vi "z_opti_rnd.vi"(0 "IP address":string="172.24.192.135", 1 "range[nm]":dbl, 3 "n":i32, 5 "Axis":string(combo), 7 "rand[t] seq [f]":bool, 9 "data":refnum<queue>, 11 "cam":refnum<queue>, 12 "error in (no error)":errorcluster) -> (4 "X":dbl[](array[numeric]), 6 "Y":dbl[](array[numeric]), 10 "Best Gaussian Fit":dbl[](array[numeric]), 14 "error out":errorcluster, 15 "center":dbl)   [LabVIEW 2017]
uses:
  <vilib>/gmath/NumericalOptimization/Nonlinear Curve Fit LM.vi
  <vilib>/gmath/NI_Gmath.lvlib
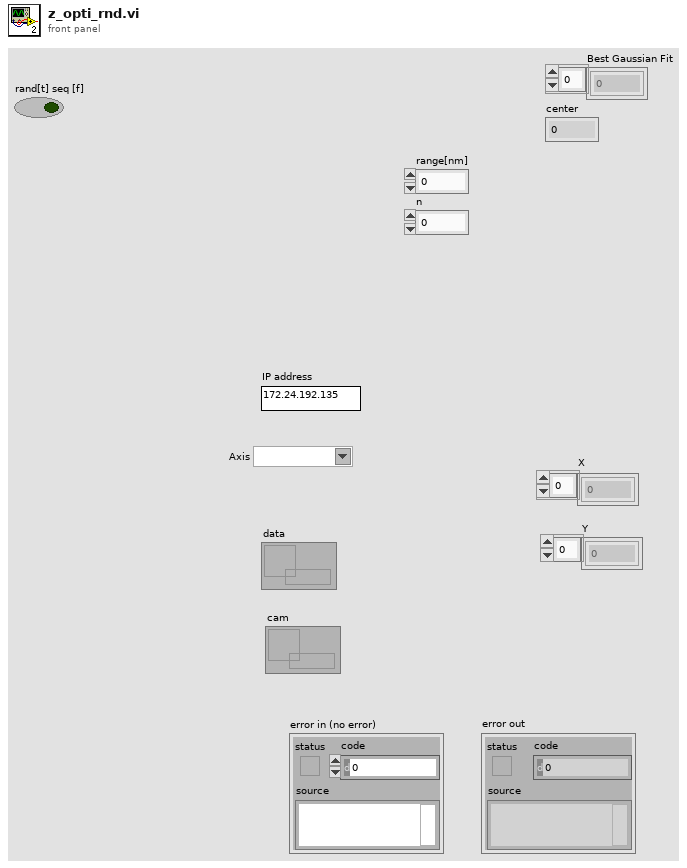
[diagram p1: front panel]
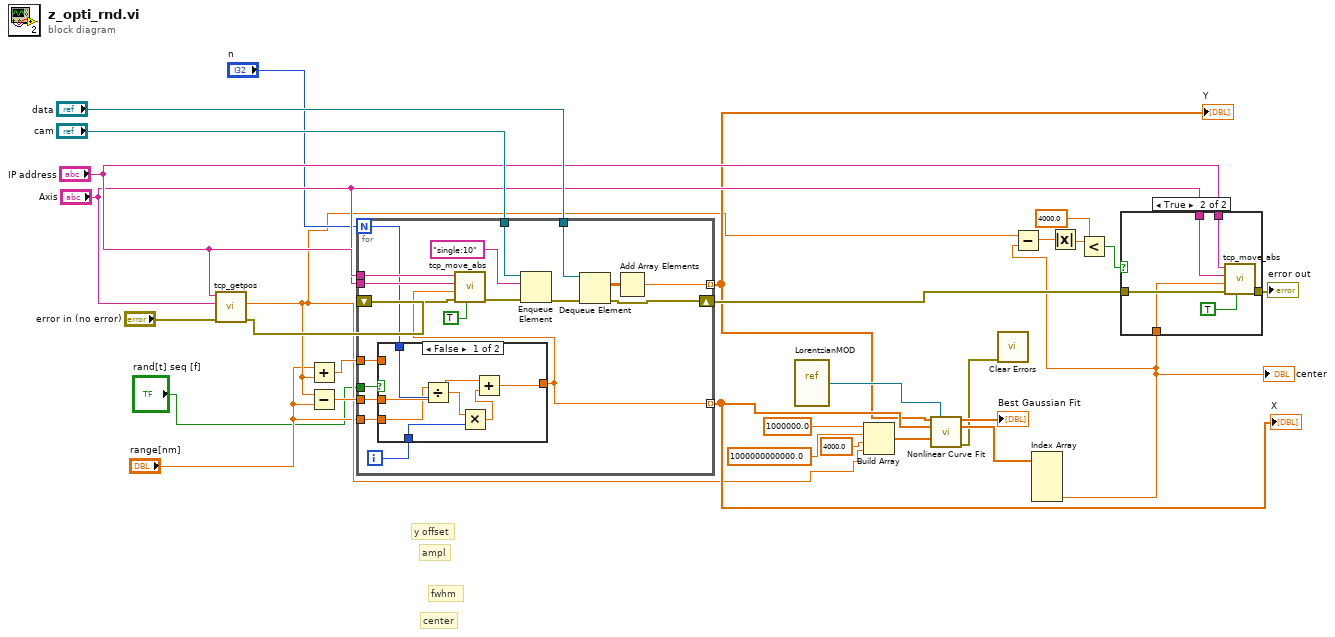
[diagram p0: block diagram]
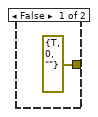
[diagram p2: hidden frame]
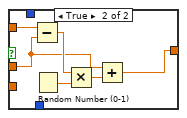
[diagram p3: hidden frame]
diagram:
  # "fwhm"
  # "ampl"
  # "center"
  # "y offset"
  n1 = call "tcp_getpos.vi"("error in (no error)"="error in (no error)", "Axis"="Axis", "IP address"="IP address") -> ("error out"=w24:errorcluster, "position"=w7:dbl)  [unwired: 6 in, 1 out]
  n2 = Add(x="range[nm]", y=w7) -> (x+y=w21:dbl)
  n3 = Subtract(x=w7, y="range[nm]") -> (x-y=w20:dbl)
  n4 = for {
    N: "n" -> [w32]
    tunnel: "Axis" -> [w48]
    tunnel: "IP address" -> [w47]
    tunnel: "cam" -> [w43]
    tunnel: "data" -> [w44]
    tunnel: [w39] -> w12 mode=indexing
    shift-right: [w37] -> w23
    shift-left: w24 -> [w38]
    tunnel: w21 -> [w36]
    tunnel: w20 -> [w35]
    tunnel: [w34] -> w17 mode=indexing
    tunnel: "range[nm]" -> [w31]
    tunnel: "rand[t] seq [f]" -> [w30]
    i -> [w33]
    n5 = case shown="False" w30 {
      tunnel: w36 -> [_ w58]
      tunnel: w35 -> [w55 w57]
      tunnel: [w54 w56] -> w34
      tunnel: w33 -> [w51 _]
      tunnel: w32 -> [w53 _]
      tunnel: w31 -> [w49 _]
      frame False {
        n6 = Divide(x=w49, y=w53) -> (x/y=w52:dbl)
        n7 = Multiply(x=w52, y=w51) -> (x*y=w50:dbl)
        n8 = Add(x=w55, y=w50) -> (x+y=w54:dbl)
      }
      frame True {
        n9 = Subtract(x=w58, y=w57) -> (x-y=w61:dbl)
        n10 = Random Number (0-1)() -> (number: 0 to 1=w60:dbl)
        n11 = Multiply(x=w61, y=w60) -> (x*y=w59:dbl)
        n12 = Add(x=w57, y=w59) -> (x+y=w56:dbl)
      }
    }
    n13 = call "tcp_move_abs.vi"("wait4motiondone"=TRUE, "error in (no error)"=w38, "destination nm/u°"=w34, "Axis"=w48, "IP address"=w47) -> ("error out"=w46:errorcluster)  [unwired: 4 in, 2 out]
    n14 = Enqueue Element(queue=w43, element="single:10", error in (no error)=w46) -> (error out=w45:errorcluster)  [unwired: 1 in, 2 out]
    n15 = Dequeue Element(queue=w44, error in (no error)=w45) -> (element=w40:dbl[][], error out=w37:errorcluster)  [unwired: 1 in, 2 out]
    n16 = Add Array Elements(numeric array=w40) -> (sum=w39:dbl)
  }
  "Y" <- w12
  "X" <- w17
  n17 = vi-ref "LorentzianMOD.vi"() -> (w18:refnum<vi>)
  n18 = Build Array(1000000.0 ("element"), 1000000000000.0 ("element"), 4000.0 ("element"), w7) -> (w14:dbl[])
  n19 = call-poly <vilib>:"Nonlinear Curve Fit.vi"("Y"=w12, "f(x,a)"=w18, "X"=w17, "initial parameters"=w14) -> ("best nonlinear fit"=→"Best Gaussian Fit":dbl[], "best fit parameters"=w10:dbl[], "error out"=w9:errorcluster)  [unwired: 6 in, 3 out]
  n20 = call <vilib>:"Clear Errors.vi"("error in (no error)"=w9) -> ()  [unwired: 5 in, 2 out]
  n21 = Index Array(array=w10) -> (element #4=w8:dbl)  [unwired: 4 in, 3 out]
  "center" <- w8
  n22 = Subtract(x=w7, y=w8) -> (x-y=w6:dbl)
  n23 = Absolute Value(x=w6) -> (abs(x)=w5:dbl)
  n24 = Less?(x=w5, y=4000.0) -> (x < y?=w3:bool)
  n25 = case shown="True" w3 {
    tunnel: "IP address" -> [_ w68]
    tunnel: "Axis" -> [_ w66]
    tunnel: w23 -> [_ w65]
    tunnel: [errorcluster {"status"=TRUE, "code"=0, "source"=""} ("error out") w64] -> w22
    tunnel: w8 -> [_ w63]
    frame False {
    }
    frame True {
      n26 = call "tcp_move_abs.vi"("wait4motiondone"=TRUE, "error in (no error)"=w65, "destination nm/u°"=w63, "Axis"=w66, "IP address"=w68) -> ("error out"=w64:errorcluster)  [unwired: 4 in, 2 out]
    }
  }
  "error out" <- w22
